vi "ploygon_vertex_array.vi"(7 "initial_angle":dbl, 8 "r":dbl=100.0, 9 "c_y":dbl=500.0, 10 "c_x":dbl=500.0, 11 "P_num":i32=6) -> (2 "Array 2":dbl[][](array[numeric]))   [LabVIEW 2016]
panel:
  in  "for array test":bool
  out "Array 3":dbl[](array[numeric])
  out "Array":dbl[](array[numeric])
  out "polygon_angle":dbl
  out "R":dbl
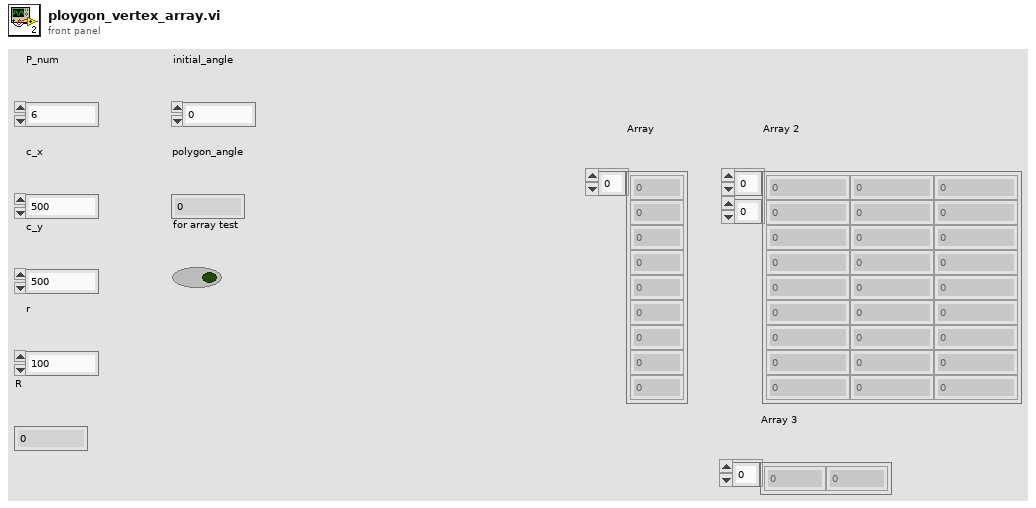
[diagram p1: front panel]
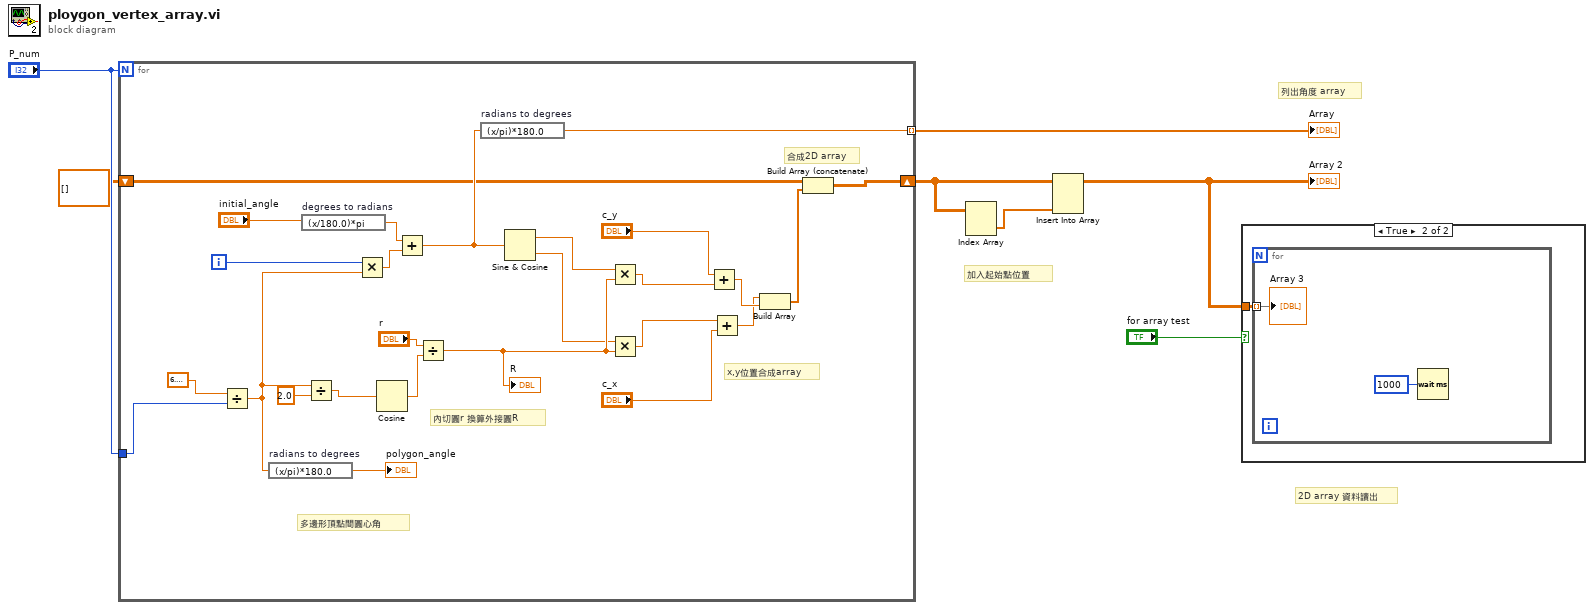
[diagram p0: block diagram]
diagram:
  # "列出角度 array"
  # "加入起始點位置"
  # "2D array 資料讀出"
  n1 = for {
    N: "P_num" -> [_]
    tunnel: "P_num" -> [w30]
    tunnel: [w17] -> w6 mode=indexing
    shift-right: [w15] -> w3
    shift-left: dbl[][] [] -> [w14]
    i -> [w28]
    # "內切圓r 換算外接圓R"
    # "多邊形頂點間圓心角"
    # "合成2D array"
    # "x,y位置合成array"
    n2 = Divide(x=6.283185307179586, y=w30) -> (x/y=w23:dbl)
    n3 = expression code="(x/pi)*180.0" "radians to degrees"(w23) -> (→"polygon_angle":dbl)
    n4 = expression code="(x/180.0)*pi" "degrees to radians"("initial_angle") -> (w25:dbl)
    n5 = Divide(x=w23, y=2.0) -> (x/y=w21:dbl)
    n6 = Multiply(x=w28, y=w23) -> (x*y=w27:dbl)
    n7 = Cosine(x=w21) -> (cos(x)=w32:dbl)
    n8 = Add(x=w25, y=w27) -> (x+y=w18:dbl)
    n9 = Divide(x="r", y=w32) -> (x/y=w24:dbl)
    "R" <- w24
    n10 = expression code="(x/pi)*180.0" "radians to degrees"(w18) -> (w17:dbl)
    n11 = Sine & Cosine(0:w18) -> (1:w19:dbl, 2:w20:dbl)
    n12 = Multiply(x=w19, y=w24) -> (x*y=w12:dbl)
    n13 = Multiply(x=w20, y=w24) -> (x*y=w11:dbl)
    n14 = Add(x="c_y", y=w12) -> (x+y=w9:dbl)
    n15 = Add(x=w11, y="c_x") -> (x+y=w8:dbl)
    n16 = Build Array(w8, w9) -> (w16:dbl[])
    n17 = Build Array (concatenate)(w14, w16) -> (w15:dbl[][])
  }
  "Array" <- w6
  n18 = Index Array(array=w3) -> (element=w2:dbl[])  [unwired: 2 in]
  n19 = Insert Into Array(array=w3, new element=w2) -> (w4:dbl[][])  [unwired: 2 in]
  "Array 2" <- w4
  n20 = case shown="True" "for array test" {
    tunnel: w4 -> [_ w34]
    frame False {
    }
    frame True {
      n21 = for {
        tunnel: w34 -> [w35] mode=indexing
        n22 = Wait (ms)(milliseconds to wait=u32 1000) -> ()  [unwired: 1 out]
        "Array 3" <- w35
      }
    }
  }
